vi "Read External Launch.vi"(8 "error in (no error)":errorcluster, 11 "NistModuleAdminBase in":refnum<class "ModuleAdminBase.lvclass">) -> (0 "error out":errorcluster, 2 "External Launch":bool, 3 "NistModuleAdminBase out":refnum<class "ModuleAdminBase.lvclass">)   [LabVIEW 2014, in "ModuleAdmin.lvlib" / "ModuleAdminBase.lvclass"]
uses:
  ModuleAdminBase.lvclass
  ModuleAdminBase.lvclass/ModuleAdminBase.ctl
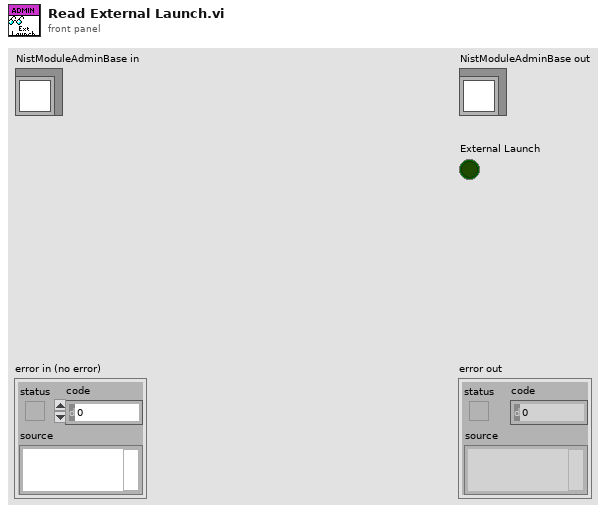
[diagram p1: front panel]
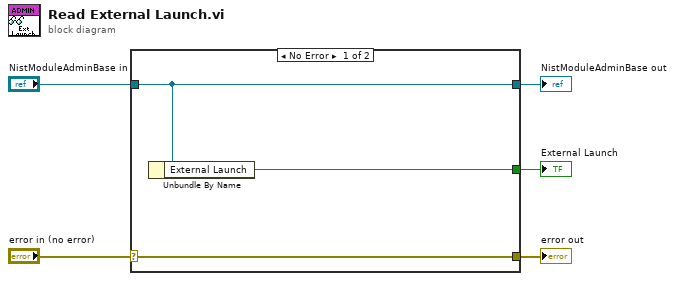
[diagram p0: block diagram]
diagram:
  n1 = case shown="No Error" "error in (no error)" {
    selector: "error in (no error)" -> [w8 w9]
    tunnel: [w8 w9] -> w4
    tunnel: [w7 w10] -> w2
    tunnel: "NistModuleAdminBase in" -> [w7 w10]
    tunnel: [w6 _] -> w1
    frame No Error {
      n2 = Unbundle By Name(w7) -> ("External Launch"=w6:bool)
    }
    frame Error {
    }
  }
  "error out" <- w4
  "NistModuleAdminBase out" <- w2
  "External Launch" <- w1
